vi "Main_Measurement.vi"(5 "error in":errorcluster) -> (19 "error out":errorcluster)   [LabVIEW 2013]
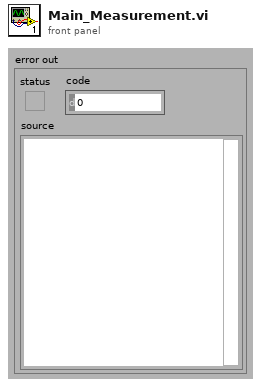
[diagram p1: front panel]
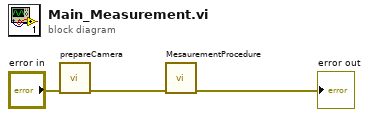
[diagram p0: block diagram]
diagram:
  n1 = call "prepareCamera.vi"("error in (no error)"="error in") -> ("error out"=w2:errorcluster)  [unwired: 10 in]
  n2 = call "MesaurementProcedure.vi"("error in (no error)"=w2) -> ("error out"=→"error out":errorcluster)  [unwired: 10 in]
